vi "Write.vi"(8 "error in (no error)":errorcluster, 9 "Variant":variant, 10 "String":string, 11 "Ethernet in":refnum<class "TCP.lvclass">) -> (0 "error out":errorcluster, 3 "Ethernet out":refnum<class "TCP.lvclass">)   [LabVIEW 2023, in "Protocols.lvlib" / "TCP.lvclass"]
uses:
  TCP.lvclass
  Protocol Parent/Protocol Parent.lvclass
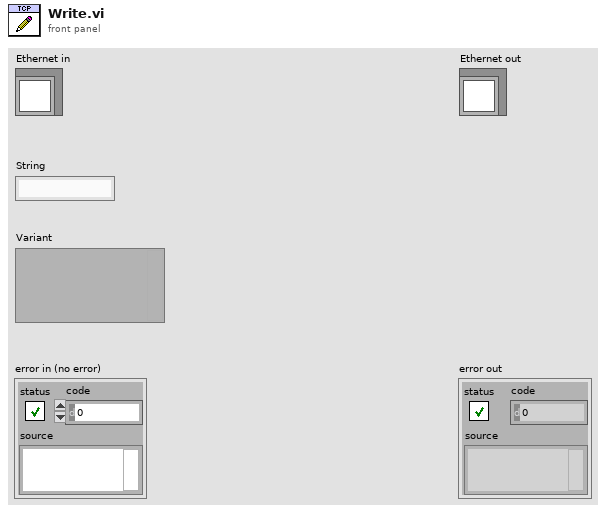
[diagram p1: front panel]
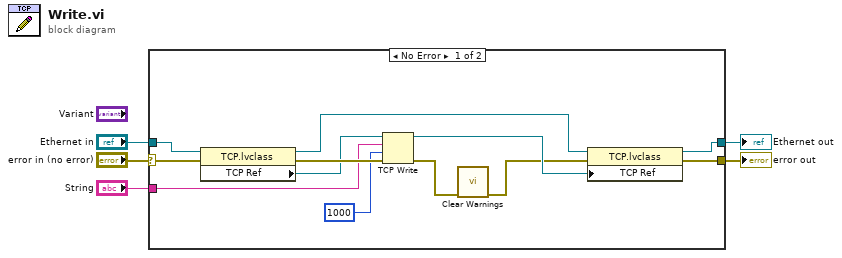
[diagram p0: block diagram]
diagram:
  n1 = case shown="No Error" "error in (no error)" {
    selector: "error in (no error)" -> [w9 w19]
    tunnel: "Ethernet in" -> [w16 w18]
    tunnel: [w12 w19] -> w4
    tunnel: [w11 w18] -> w3
    tunnel: "String" -> [w10 _]
    frame No Error {
      n2 = property class="TCP.lvclass"(reference=w16, error in=w9) -> (reference out=w14:refnum<class "TCP.lvclass">, error out=w17:errorcluster, "TCP Ref"=w15:refnum<k5>)
      n3 = TCP Write(connection ID=w15, data in=w10, error in (no error)=w17, 9:1000 ("timeout ms (25000)")) -> (connection ID out=w13:refnum<k5>, error out=w7:errorcluster)  [unwired: 1 out]
      n4 = call "Clear Warnings.vi"("error in (no error)"=w7) -> ("error out"=w6:errorcluster)  [unwired: 10 in]
      n5 = property class="TCP.lvclass"(reference=w14, error in=w6, "TCP Ref"=w13) -> (reference out=w11:refnum<class "TCP.lvclass">, error out=w12:errorcluster)
    }
    frame Error {
    }
  }
  "error out" <- w4
  "Ethernet out" <- w3
